vi "MEMR-Plot Analysis Band.vi"(0 "XYGraph in":refnum<vi>, 7 "Fpeak":dbl[](array[numeric]), 11 "error in (no error)":errorcluster) -> (15 "error out":errorcluster)   [LabVIEW 2020]
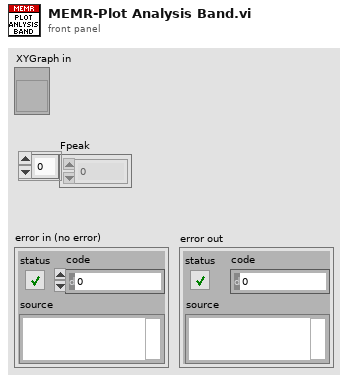
[diagram p1: front panel]
types:
  T1 = typedef "LVRectTypeDef.ctl" = cluster{"Left":i16, "Top":i16, "Right":i16, "Bottom":i16}
  T2 = typedef "LVPoint32TypeDef.ctl" = cluster{"Horizontal":i32, "Vertical":i32}
  T3 = cluster{"Width":u16, "Style":enum32{"Solid", "Dash", "Dot", "DashDot", "DashDotDot"}}
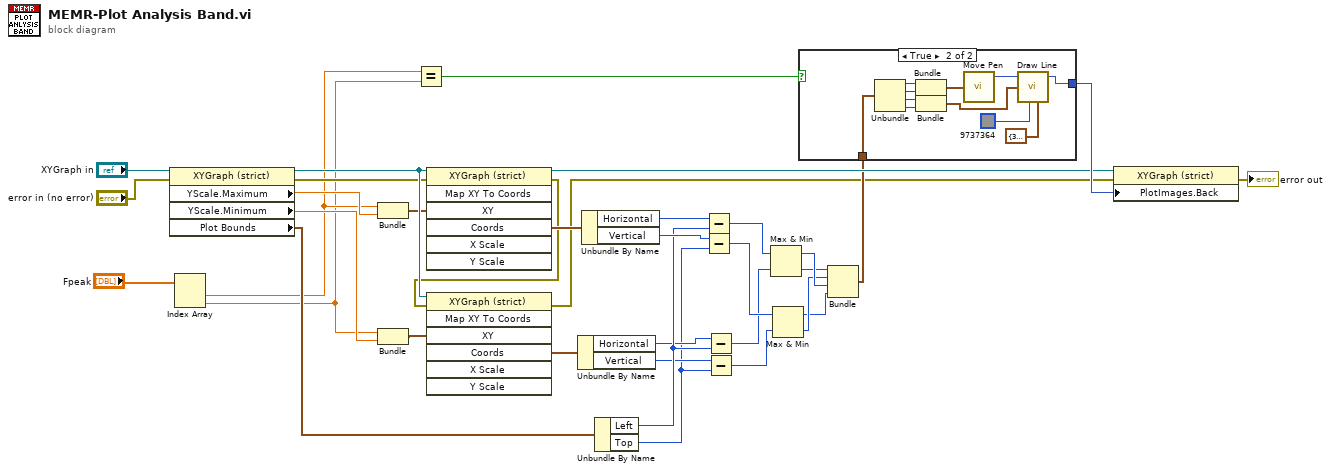
[diagram p0: block diagram]
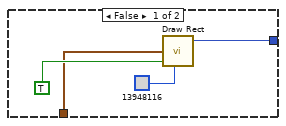
[diagram p2: hidden frame]
diagram:
  n1 = property on="Property Node" class="XYGraph (strict)"(reference="XYGraph in", error in="error in (no error)") -> (reference out=w35:refnum<vi>, error out=w29:errorcluster, "YScale.Maximum"=w33:dbl, "YScale.Minimum"=w34:dbl, "Plot Bounds"=w30:T1)
  n2 = Index Array(array="Fpeak") -> (element #1=w5:dbl, element #2=w4:dbl)  [unwired: 2 in]
  n3 = Bundle("Numeric"=w5, "YScale.Maximum"=w33) -> (w26:cluster{"Numeric":dbl, "YScale.Maximum":dbl})  [unwired: 1 in]
  n4 = Bundle("Numeric"=w4, "YScale.Minimum"=w34) -> (w25:cluster{"Numeric":dbl, "YScale.Minimum":dbl})  [unwired: 1 in]
  n5 = Equal?(x=w5, y=w4) -> (x = y?=w3:bool)
  n6 = invoke on="Invoke Node" class="XYGraph (strict)" method="Map XY To Coords"(reference=w35, error in=w29, "XY"=w26) -> (reference out=w28:refnum<vi>, error out=w2:errorcluster, "Coords"=w21:T2)  [unwired: 4 in, 4 out]
  n7 = invoke on="Invoke Node" class="XYGraph (strict)" method="Map XY To Coords"(reference=w35, error in=w2, "XY"=w25) -> (error out=w1:errorcluster, "Coords"=w20:T2)  [unwired: 4 in, 5 out]
  n8 = Unbundle By Name(w20) -> ("Horizontal"=w12:i32, "Vertical"=w10:i32)
  n9 = Unbundle By Name(w21) -> ("Horizontal"=w17:i32, "Vertical"=w15:i32)
  n10 = Unbundle By Name(w30) -> ("Left"=w13:i16, "Top"=w9:i16)
  n11 = Subtract(x=w17, y=w13) -> (x-y=w16:i32)
  n12 = Subtract(x=w15, y=w9) -> (x-y=w14:i32)
  n13 = Subtract(x=w12, y=w13) -> (x-y=w11:i32)
  n14 = Subtract(x=w10, y=w9) -> (x-y=w8:i32)
  n15 = Max & Min(x=w16, y=w11) -> (max(x,y)=w24:i32, min(x,y)=w22:i32)
  n16 = Max & Min(x=w14, y=w8) -> (max(x,y)=w18:i32, min(x,y)=w23:i32)
  n17 = Bundle(w22, w23, w24, w18) -> (w19:cluster{i32, i32, i32, i32})  [unwired: 1 out]
  n18 = case shown="True" w3 {
    tunnel: [w39 w44] -> w32
    tunnel: w19 -> [w37 w50]
    frame False {
      n19 = call <vilib>:"Draw Rect.vi"("rect"=w37, "fill?(F)"=TRUE, "color(black)"=u32 13948116) -> ("new picture"=w39:picture)  [unwired: 2 in, 4 out]
    }
    frame True {
      n20 = Unbundle(w50) -> (w49:i32, w48:i32, w46:i32, w45:i32)
      n21 = Bundle(w49, w48) -> (w47:cluster{i32, i32})  [unwired: 1 in]
      n22 = Bundle(w46, w45) -> (w42:cluster{i32, i32})  [unwired: 1 in]
      n23 = call <vilib>:"Move Pen.vi"("new position"=w47) -> ("new picture"=w43:picture)  [unwired: 4 in]
      n24 = call <vilib>:"Draw Line.vi"("picture"=w43, "end point"=w42, "color(black)"=u32 9737364, "pen"=T3 {"Width"=3, "Style"=enum."Solid"}) -> ("new picture"=w44:picture)  [unwired: 5 in]
    }
  }
  n25 = property on="Property Node" class="XYGraph (strict)"(reference=w28, error in=w1, "PlotImages.Back"=w32) -> (error out=→"error out":errorcluster)  [unwired: 1 out]
